vi "MDAQ_ThresholdHelper.vi"(10 "Input Array":u32[](array[numeric]), 11 "WaveformGraph in":refnum<vi>) -> ()   [LabVIEW 2021]
uses:
  <vilib>/Analysis/baseanly.llb/Mean (DBL).vi
  <vilib>/Analysis/NI_AALBase.lvlib
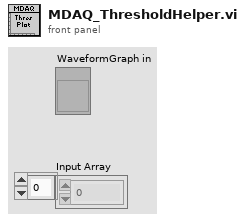
[diagram p1: front panel]
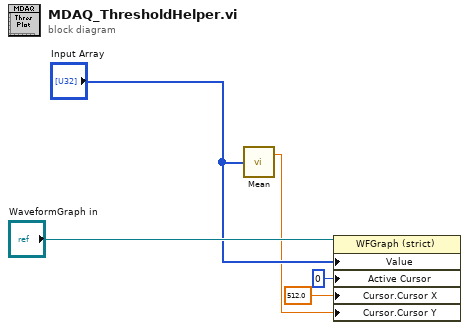
[diagram p0: block diagram]
diagram:
  n1 = call-poly <vilib>:"Mean.vi"("X"="Input Array") -> ("mean"=w1:dbl)  [unwired: 1 out]
  n2 = property class="WFGraph (strict)"(reference="WaveformGraph in", "Value"="Input Array", "Active Cursor"=u32 0, "Cursor.Cursor X"=512.0 ("Cursor.Cursor Position:Cursor X"), "Cursor.Cursor Y"=w1) -> ()  [unwired: 1 in, 2 out]
